vi "Front Panel Image to IMAQ.vi"() -> ()   [LabVIEW 2020]
uses:
  Instance           1 33Saved   Front Panel Image to IMAQ .vi
panel:
  out "Image":T1(plugin-control)
  out "Sine":dynamicdata(graph)
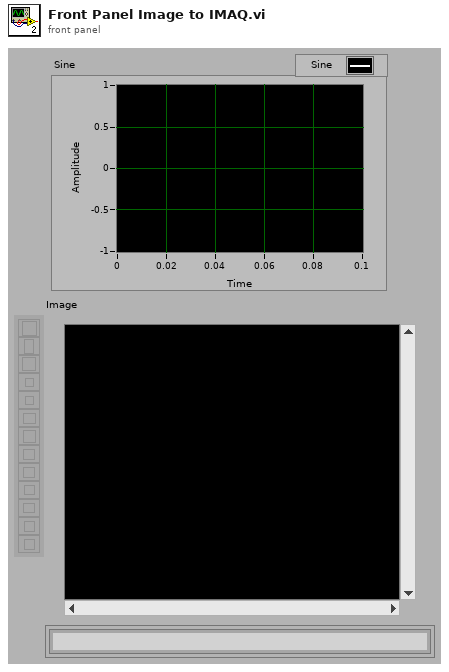
[diagram p1: front panel]
types:
  T1 = typedef "IMAQ Image.ctl" = refnum<image>
  T2 = typedef "Image Type" = u32
  T3 = typedef "imagedata.ctl" = cluster{"image type":i32, "image depth":i32, "image":u8[], "mask":u8[], "colors":u32[], "Rectangle":cluster{"left":i16, "top":i16, "right":i16, "bottom":i16}}
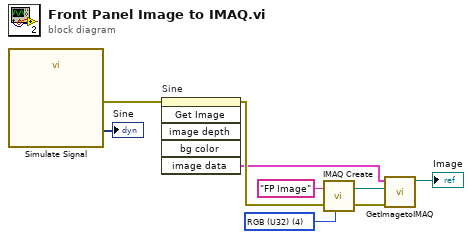
[diagram p0: block diagram]
diagram:
  w6 = T2 4 items=["Grayscale (U8)", "Grayscale (I16)", "Grayscale (SGL)", "Complex (CSG)", "RGB (U32)", "HSL (U32)", "RGB (U64)", "Grayscale (U16)"] ("Image Type")
  n1 = call "Simulate Signal"() -> ("Sine"=→"Sine":dynamicdata, "error out"=w8:errorcluster)  [unwired: 14 in]
  n2 = invoke on="Sine" class="WFGraph (strict)" method="Get Image"(error in=w8) -> (error out=w5:errorcluster, "image data"=w2:T3)  [unwired: 5 in, 4 out]
  n3 = call "IMAQ Create"("Image Name"="FP Image", "Image Type"=w6, "error in (no error)"=w5) -> ("New Image"=w4:T1, "error out"=w3:errorcluster)  [unwired: 2 in]
  n4 = call "GetImagetoIMAQ.vi"("error in (no error)"=w3, "Image Src"=w4, "Image Data"=w2) -> ("Image Out"=→"Image":T1)  [unwired: 7 in, 1 out]
